vi "tm3samp_functions.vi"() -> ()   [LabVIEW 2012]
panel:
  out "Image":u16[][](graph)
  in  "Snap":bool
  in  "Parameter":i32(ring)
  in  "Text Value":dbl(ring)
  in  "Value":dbl(slide) min=1.0 max=5.0 scale=1.0..5.0
  out "error out":errorcluster
  in  "stop":bool
  # "This example shows a way you can access\nmany of the functions available to the camera and see how they affect the captured image."
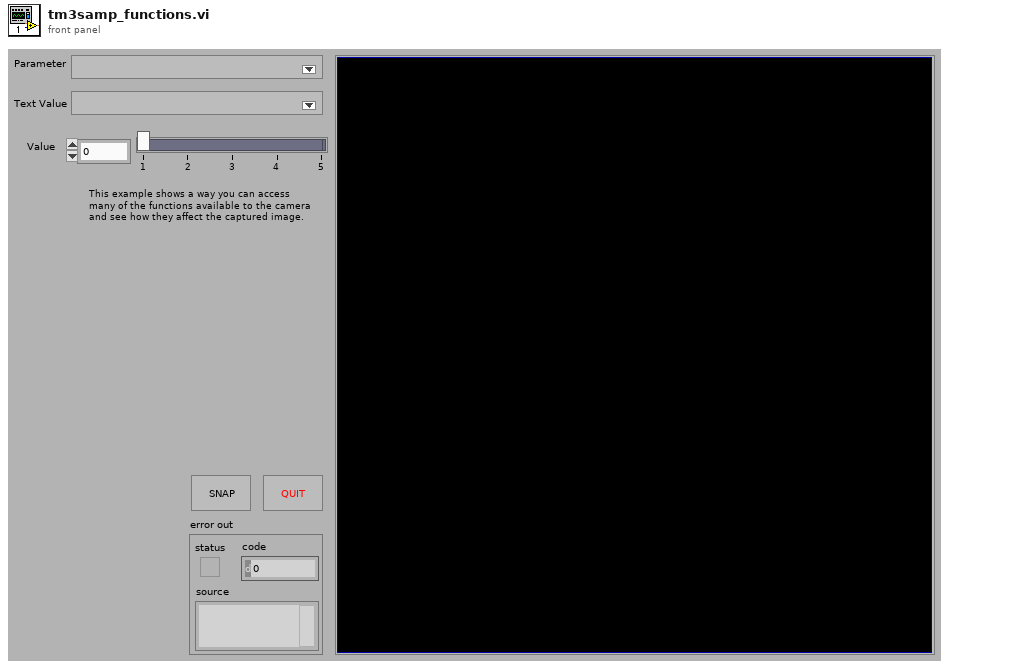
[diagram p1: front panel]
types:
  T1 = enum8{"Enabled", "Disabled", "Disabled and Grayed Out"}
  T2 = cluster{"Function Name":string, "Function ID":dbl}[]
  T3 = cluster{"width":u32, "height":u32, "datatype":u32}
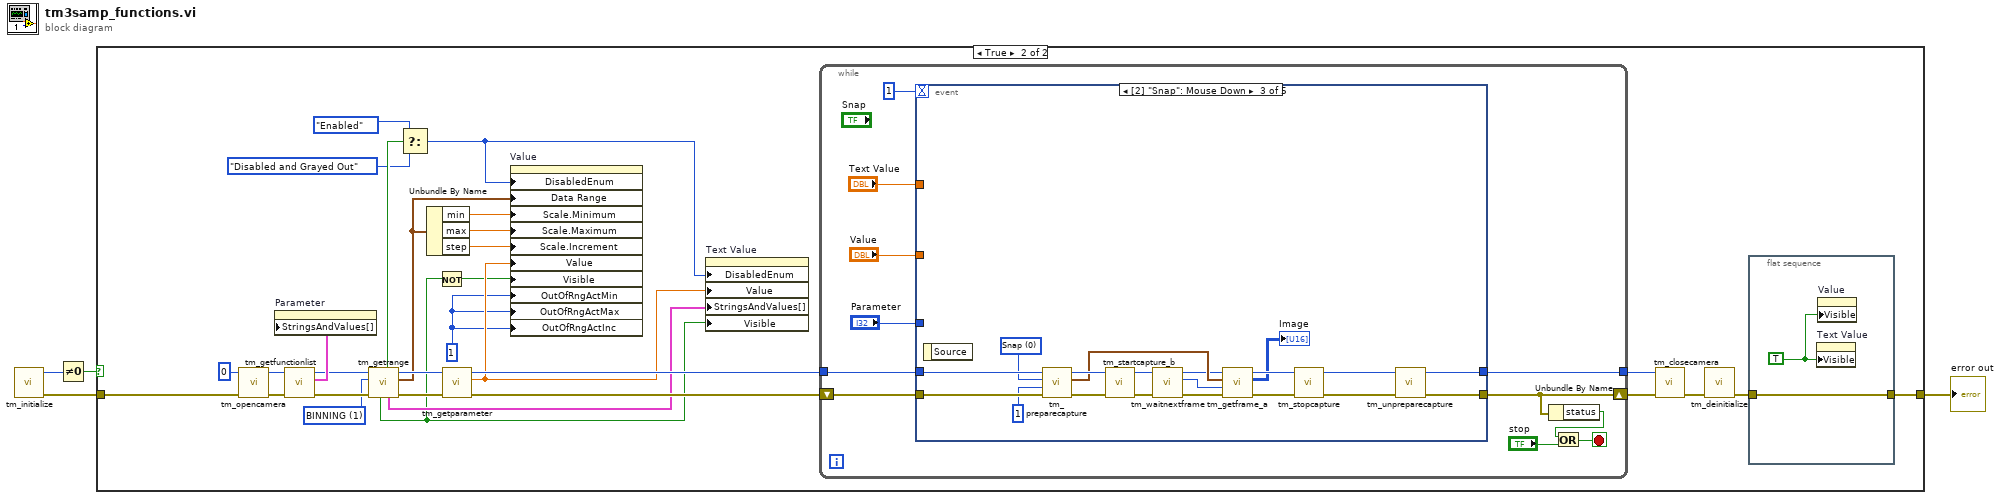
[diagram p0: block diagram]
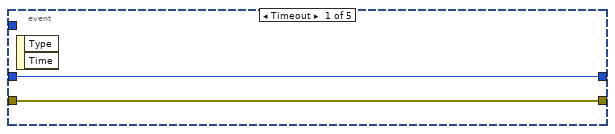
[diagram p3: hidden frame]
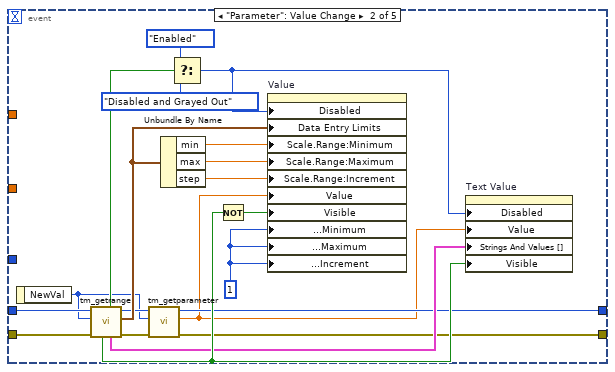
[diagram p4: hidden frame]
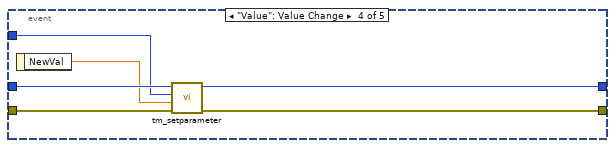
[diagram p5: hidden frame]
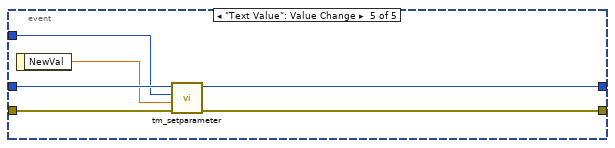
[diagram p6: hidden frame]
diagram:
  n1 = call <userlib>:"tm_initialize.vi"() -> ("error out"=w2:errorcluster, "Number Of Cameras"=w4:u32)  [unwired: 10 in]
  n2 = Not Equal To 0?(x=w4) -> (x != 0?=w3:bool)
  n3 = case shown="True" w3 {
    tunnel: [w5 w29] -> w1
    tunnel: w2 -> [w5 w35]
    frame False {
    }
    frame True {
      w16 = 1 items=["BINNING"=1, "BITS PER CHANNEL"=2, "ACTIVE VIEW INDEX"=3, "CCD MODE"=4, "SENSOR MODE"=5, "READOUT MODE"=6, "EXPOSURE TIME"=7, "CONTRAST GAIN"=8, "CONTRAST OFFSET"=9, "LIGHT MODE"=10, "SENSITIVITY"=11, "WHITE BALANCE"=12, "PHOTON IMAGING MODE"=13, "HIGH DYNAMIC RANGE MODE"=14, "TRIGGER SOURCE"=15, "TRIGGER ACTIVE"=16, "TRIGGER MODE"=17, "TRIGGER POLARITY"=18, "TRIGGER GLOBAL EXPOSURE"=19, "FIRST TRIGGER BEHAVIOR"=20, "TRIGGER TIMES"=21, "OUTPUT TRIGGER POLARITY"=22, "OUTPUT TRIGGER DELAY"=23, "OUTPUT TRIGGER PERIOD"=24, "TEMPERATURE"=25, "TEMPERATURE TARGET"=26, "SENSOR COOLER FAN"=27, "MECHANICAL SHUTTER"=28, "BACK FOCUS POSITION"=29, "FRAMEBUNDLE MODE"=30, "FRAMEBUNDLE NUMBER"=31] ("Parameter")
      w6 = u8 1 ("Out Of Range Action:Increment")
      n4 = call <userlib>:"tm_opencamera.vi"("error in (no error)"=w35, "Camera Index"=u32 0) -> ("error out"=w32:errorcluster, "Handle out"=w33:u32)  [unwired: 8 in]
      n5 = call <userlib>:"tm_getfunctionlist.vi"("error in (no error)"=w32, "Handle in"=w33) -> ("error out"=w19:errorcluster, "Function List"=w31:T2, "Handle out"=w20:u32)  [unwired: 7 in]
      n6 = property on="Parameter" class="Ring (strict)"("StringsAndValues[]"=w31) -> ()  [unwired: 2 in, 2 out]
      n7 = call <userlib>:"tm_getrange.vi"("error in (no error)"=w19, "Parameter"=w16, "Handle in"=w20) -> ("error out"=w21:errorcluster, "Range"=w7:cluster{"min":dbl, "max":dbl, "step":dbl}, "Handle out"=w22:u32, "Value Names"=w15:cluster{"Name":string, "Value":dbl}[], "Writable"=w25:bool, "Text Values"=w14:bool)  [unwired: 2 in, 1 out]
      n8 = Select(t=T1."Enabled" ("Disabled"), s=w25, f=T1."Disabled and Grayed Out" ("Disabled")) -> (s? t:f=w13:T1)
      n9 = Unbundle By Name(w7) -> ("min"=w12:dbl, "max"=w11:dbl, "step"=w10:dbl)
      n10 = Not(x=w14) -> (.not. x?=w8:bool)
      n11 = call <userlib>:"tm_getparameter.vi"("error in (no error)"=w21, "Handle in"=w22) -> ("error out"=w17:errorcluster, "Value out"=w9:dbl, "Handle out"=w18:u32)  [unwired: 7 in]
      n12 = property on="Value" class="Slide (strict)"("DisabledEnum"=w13, "Data Range"=w7, "Scale.Minimum"=w12, "Scale.Maximum"=w11, "Scale.Increment"=w10, "Value"=w9, "Visible"=w8, "OutOfRngActMin"=w6, "OutOfRngActMax"=w6, "OutOfRngActInc"=w6) -> ()  [unwired: 2 in, 2 out]
      n13 = property on="Text Value" class="Ring (strict)"("DisabledEnum"=w13, "Value"=w9, "StringsAndValues[]"=w15, "Visible"=w14) -> ()  [unwired: 2 in, 2 out]
      n14 = while {
        tunnel: w18 -> [w44]
        tunnel: [w42] -> w27
        shift-right: [w41] -> w28
        shift-left: w17 -> [w45]
        stop <- w46 stop-if-true
        n15 = event shown="[2] \"Snap\": Mouse Down" {
          selector: _ -> [_ _ _ _ _]
          dyn-events: _ -> [_ _ _ _ _]
          timeout: 1 -> [_ _ _ _ _]
          tunnel: w45 -> [w50 w70 w88 w95 w101]
          tunnel: w44 -> [w49 w69 w89 w94 w100]
          tunnel: [w49 w53 w78 w93 w99] -> w42
          tunnel: [w50 w51 w77 w92 w98] -> w41
          tunnel: "Parameter" -> [_ _ _ w91 w97]
          tunnel: "Value" -> [_ _ _ _ _]
          tunnel: "Text Value" -> [_ _ _ _ _]
          event Timeout {
            n16 = event-data() -> ()  [unwired: 1 in, 2 out]
          }
          event "Parameter": Value Change {
            w62 = u8 1 ("Out Of Range Action:Increment")
            n17 = event-data() -> ("NewVal"=w55:i32)  [unwired: 1 in]
            n18 = call <userlib>:"tm_getrange.vi"("error in (no error)"=w70, "Parameter"=w55, "Handle in"=w69) -> ("error out"=w54:errorcluster, "Range"=w67:cluster{"min":dbl, "max":dbl, "step":dbl}, "Handle out"=w56:u32, "Value Names"=w60:cluster{"Name":string, "Value":dbl}[], "Writable"=w68:bool, "Text Values"=w61:bool)  [unwired: 2 in, 1 out]
            n19 = call <userlib>:"tm_getparameter.vi"("error in (no error)"=w54, "Parameter"=w55, "Handle in"=w56) -> ("error out"=w51:errorcluster, "Value out"=w52:dbl, "Handle out"=w53:u32)  [unwired: 6 in]
            n20 = Unbundle By Name(w67) -> ("min"=w66:dbl, "max"=w65:dbl, "step"=w64:dbl)
            n21 = Select(t=T1."Enabled" ("Disabled"), s=w68, f=T1."Disabled and Grayed Out" ("Disabled")) -> (s? t:f=w59:T1)
            n22 = Not(x=w61) -> (.not. x?=w63:bool)
            n23 = property on="Value" class="Slide (strict)"("Disabled"=w59, "Data Entry Limits"=w67, "Scale.Range:Minimum"=w66, "Scale.Range:Maximum"=w65, "Scale.Range:Increment"=w64, "Value"=w52, "Visible"=w63, "Response to Value Outside Limits:Minimum"=w62, "Response to Value Outside Limits:Maximum"=w62, "Response to Value Outside Limits:Increment"=w62) -> ()  [unwired: 2 in, 2 out]
            n24 = property on="Text Value" class="Ring (strict)"("Disabled"=w59, "Value"=w52, "Strings And Values []"=w60, "Visible"=w61) -> ()  [unwired: 2 in, 2 out]
          }
          event "Snap": Mouse Down {
            w87 = 0 items=["Snap", "Sequence"] ("Capture mode")
            n25 = event-data() -> ()  [unwired: 1 in, 1 out]
            n26 = call <userlib>:"tm_preparecapture.vi"("error in (no error)"=w88, "Frames"=1, "Capture mode"=w87, "Handle in"=w89) -> ("error out"=w85:errorcluster, "Buffer"=w83:T3, "Handle out"=w84:u32)  [unwired: 4 in, 1 out]
            n27 = call <userlib>:"tm_startcapture_b.vi"("error in (no error)"=w85, "Handle in"=w84) -> ("error out"=w75:errorcluster, "Handle out"=w76:u32)  [unwired: 8 in]
            n28 = call <userlib>:"tm_waitnextframe.vi"("error in (no error)"=w75, "Handle in"=w76) -> ("error out"=w73:errorcluster, "Frame Index"=w72:i32, "Handle out"=w74:u32)  [unwired: 6 in, 1 out]
            n29 = call <userlib>:"tm_getframe_a.vi"("error in (no error)"=w73, "Frame Index"=w72, "Buffer"=w83, "Handle in"=w74) -> ("error out"=w81:errorcluster, "Data 16"=→"Image":u16[][], "Handle out"=w82:u32)  [unwired: 3 in, 2 out]
            n30 = call <userlib>:"tm_stopcapture.vi"("error in (no error)"=w81, "Handle in"=w82) -> ("error out"=w80:errorcluster, "Handle out"=w79:u32)  [unwired: 8 in]
            n31 = call <userlib>:"tm_unpreparecapture.vi"("error in (no error)"=w80, "Handle in"=w79) -> ("error out"=w77:errorcluster, "Handle out"=w78:u32)  [unwired: 8 in]
          }
          event "Value": Value Change {
            n32 = event-data() -> ("NewVal"=w90:dbl)  [unwired: 1 in]
            n33 = call <userlib>:"tm_setparameter.vi"("error in (no error)"=w95, "Value in"=w90, "Parameter"=w91, "Handle in"=w94) -> ("error out"=w92:errorcluster, "Handle out"=w93:u32)  [unwired: 6 in]
          }
          event "Text Value": Value Change {
            n34 = event-data() -> ("NewVal"=w96:dbl)  [unwired: 1 in]
            n35 = call <userlib>:"tm_setparameter.vi"("error in (no error)"=w101, "Value in"=w96, "Parameter"=w97, "Handle in"=w100) -> ("error out"=w98:errorcluster, "Handle out"=w99:u32)  [unwired: 6 in]
          }
        }
        n36 = Unbundle By Name(w41) -> ("status"=w47:bool)
        n37 = Or(x=w47, y="stop") -> (x .or. y?=w46:bool)
      }
      n38 = call <userlib>:"tm_closecamera.vi"("error in (no error)"=w28, "Handle in"=w27) -> ("error out"=w34:errorcluster)  [unwired: 9 in]
      n39 = call <userlib>:"tm_deinitialize.vi"("error in (no error)"=w34) -> ("error out"=w30:errorcluster)  [unwired: 10 in]
      n40 = flat-sequence {
        tunnel: w30 -> [w37]
        tunnel: [w37] -> w29
        frame #0 {
          w36 = TRUE
          n41 = property on="Text Value" class="Ring (strict)"("Visible"=w36) -> ()  [unwired: 2 in, 2 out]
          n42 = property on="Value" class="Slide (strict)"("Visible"=w36) -> ()  [unwired: 2 in, 2 out]
        }
      }
    }
  }
  "error out" <- w1
